vi "Compressor.vi"(11 "Enum":enum16{"Start", "Run", "End"}(ring)) -> ()   [LabVIEW 2012]
uses:
  TypeDefs/PWM Module 1.ctl
  <vilib>/Rock Robotics/SystemInterfaces/Typedef/FPGA_TypedefDigitalModule.ctl
  <vilib>/Rock Robotics/SystemInterfaces/DIO/FPGA_DIOPWMChannel.ctl
  <vilib>/Rock Robotics/SystemInterfaces/DIO/FPGA_DIORelayChannel.ctl
  TypeDefs/Digital Module 1.ctl
  <vilib>/Rock Robotics/SystemInterfaces/DIO/FPGA_DIOChannel.ctl
  <vilib>/Rock Robotics/WPI/Relay/WPI_RelayDirection.ctl
  <vilib>/Rock Robotics/WPI/Relay/WPI_RelayValue.ctl
panel:
  in  "Digital Module A":T1={"Module"=enum."Digital Module 1", "Base Limit Switch"=enum."DIO 1", "Top Limit Switch"=enum."DIO 2", "Dummy Limit Switch"=enum."DIO 3", "Compressor Switch"=enum."DIO 4", "Unassigned"=enum."DIO 5", "Unassigned"=enum."DIO 6", "Unassigned"=enum."DIO 7", "Unassigned"=enum."DIO 8", "Unassigned"=enum."DIO 9", "Unassigned"=enum."DIO 10", "Unassigned"=enum."DIO 11", "Unassigned"=enum."DIO 12", "Unassigned"=enum."DIO 13", "Unassigned"=enum."DIO 14"}
  in  "PWM Module (DIO A)":T4={"Module"=enum."Digital Module 1", "Shooter"=enum."PWM 1", "Right Drive"=enum."PWM 2", "Arm"=enum."PWM 3", "Left Drive"=enum."PWM 4", "Compress"=enum."PWM 5", "Unassigned"=enum."PWM 6", "Unassigned"=enum."PWM 7", "Unassigned"=enum."PWM 8", "Unassigned"=enum."PWM 9", "Unassigned"=enum."PWM 10", "Loader"=enum."Relay 1", "Compressor"=enum."Relay 2", "Unassigned"=enum."Relay 3", "Unassigned"=enum."Relay 4", "Unassigned"=enum."Relay 5", "Unassigned"=enum."Relay 6", "Unassigned"=enum."Relay 7", "Unassigned "=enum."Relay 8"}
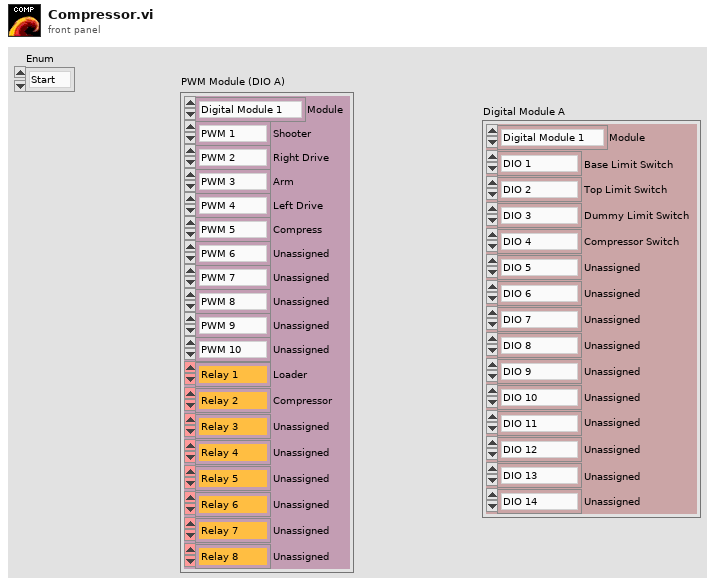
[diagram p1: front panel]
types:
  T1 = typedef "Digital Module 1.ctl" = cluster{"Module":T2, "Base Limit Switch":T3, "Top Limit Switch":T3, "Dummy Limit Switch":T3, "Compressor Switch":T3, "Unassigned":T3, "Unassigned":T3, "Unassigned":T3, "Unassigned":T3, "Unassigned":T3, "Unassigned":T3, "Unassigned":T3, "Unassigned":T3, "Unassigned":T3, "Unassigned":T3}
  T2 = typedef "FPGA_TypedefDigitalModule.ctl" = enum16{"Digital Module 1", "Digital Module 2"}
  T3 = typedef "FPGA_DIOChannel.ctl" = enum8{"DIO 1", "DIO 2", "DIO 3", "DIO 4", "DIO 5", "DIO 6", "DIO 7", "DIO 8", "DIO 9", "DIO 10", "DIO 11", "DIO 12", "DIO 13", "DIO 14", "Invalid"}
  T4 = typedef "PWM Module 1.ctl" = cluster{"Module":T2, "Shooter":T5, "Right Drive":T5, "Arm":T5, "Left Drive":T5, "Compress":T5, "Unassigned":T5, "Unassigned":T5, "Unassigned":T5, "Unassigned":T5, "Unassigned":T5, "Loader":T6, "Compressor":T6, "Unassigned":T6, "Unassigned":T6, "Unassigned":T6, "Unassigned":T6, "Unassigned":T6, "Unassigned ":T6}
  T5 = typedef "FPGA_DIOPWMChannel.ctl" = enum8{"PWM 1", "PWM 2", "PWM 3", "PWM 4", "PWM 5", "PWM 6", "PWM 7", "PWM 8", "PWM 9", "PWM 10", "Invalid"}
  T6 = typedef "FPGA_DIORelayChannel.ctl" = enum8{"Relay 1", "Relay 2", "Relay 3", "Relay 4", "Relay 5", "Relay 6", "Relay 7", "Relay 8", "Invalid"}
  T7 = typedef "WPI_RelayDirection.ctl" = enum16{"Both directions", "Forward only", "Reverse only"}
  T8 = typedef "WPI_RelayValue.ctl" = enum16{"Off", "On", "Forward", "Reverse"}
  T9 = typedef "WPI_RelayDevRef.ctl" = cluster{"DevStatus":errorcluster, "Relay Channel":T6, "Digital Module":T2, "Relay Direction":T7}
  T10 = typedef "WPI_DigitalInputDevRef.ctl" = cluster{"DevStatus":errorcluster, "DIO Channel":T3, "Digital Module":T2}
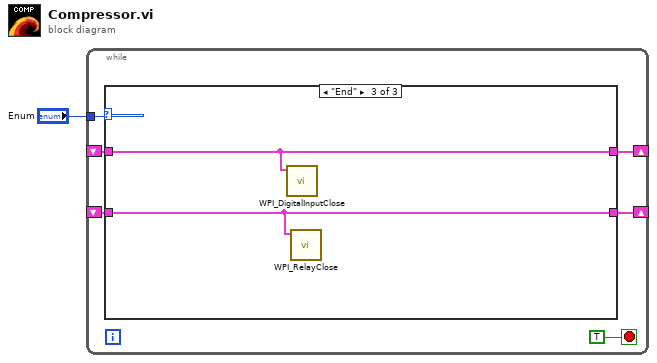
[diagram p0: block diagram]
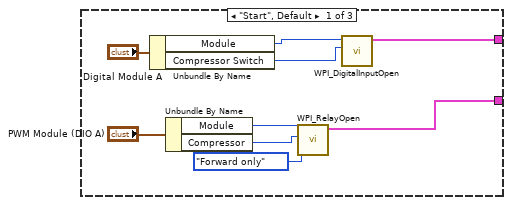
[diagram p2: hidden frame]
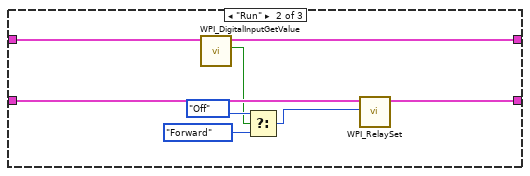
[diagram p3: hidden frame]
diagram:
  n1 = while {
    tunnel: "Enum" -> [w6]
    shift-right: [w5] -> _
    shift-left: _ -> [w4]
    shift-right: [w3] -> _
    shift-left: _ -> [w2]
    stop <- TRUE stop-if-true
    n2 = case shown="\"End\"" w6 {
      tunnel: [w8 w21 w26] -> w5
      tunnel: w4 -> [_ w22 w26]
      tunnel: [w9 w23 w25] -> w3
      tunnel: w2 -> [_ w24 w25]
      frame "Start", Default {
        n3 = Unbundle By Name("Digital Module A") -> ("Module"=w11:T2, "Compressor Switch"=w10:T3)
        n4 = Unbundle By Name("PWM Module (DIO A)") -> ("Module"=w14:T2, "Compressor"=w13:T6)
        n5 = call <vilib>:"WPI_RelayOpen.vi"("Relay Direction"=WPI_RelayDirection."Forward only", "Relay Channel"=w13, "Digital Module (Module 1)"=w14) -> ("RelayDevRef"=w8:T9)  [unwired: 7 in, 1 out]
        n6 = call <vilib>:"WPI_DigitalInputOpen.vi"("DIO Channel"=w10, "Digital Module (Module 1)"=w11) -> ("DigitalInputDevRef"=w9:T10)  [unwired: 8 in, 1 out]
      }
      frame "Run" {
        n7 = call <vilib>:"WPI_DigitalInputGetValue.vi"("DigitalInputDevRef"=w24) -> ("Value"=w19:bool, "DigitalInputDevRef"=w23:T10)  [unwired: 8 in, 1 out]
        n8 = Select(t=WPI_RelayValue."Off" ("RelayValue"), s=w19, f=WPI_RelayValue."Forward") -> (s? t:f=w17:T8)
        n9 = call <vilib>:"WPI_RelaySet.vi"("RelayValue"=w17, "RelayDevRef"=w22) -> ("RelayDevRef"=w21:T9)  [unwired: 8 in, 1 out]
      }
      frame "End" {
        n10 = call <vilib>:"WPI_DigitalInputClose.vi"("DigitalInputDevRef"=w25) -> ()  [unwired: 10 in, 1 out]
        n11 = call <vilib>:"WPI_RelayClose.vi"("RelayDevRef"=w26) -> ()  [unwired: 10 in, 1 out]
      }
    }
  }
